vi "Psych Chart Look-up BY HR.vi"(0 "Humidity Ratio [-]":dbl=72.0, 5 "Air Pressure [psia]":dbl=14.7, 7 "1st known value":dbl=55.0, 12 "1st Known Index":u16(ring) items=["DB", "WB", "RH", "HR", "Gr", "Vol", "h", "Dp"]) -> (8 "Output Array":dbl[](array[numeric]))   [LabVIEW 2020]
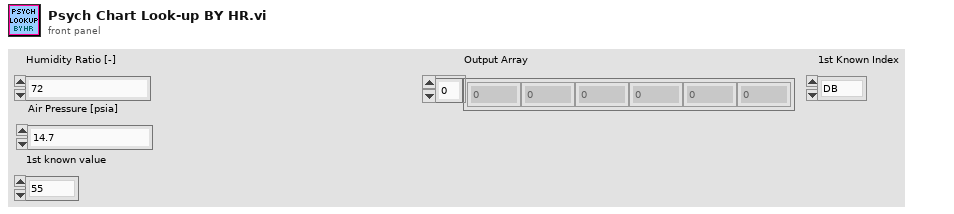
[diagram p1: front panel]
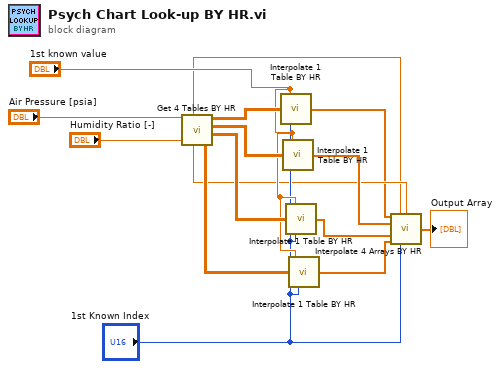
[diagram p0: block diagram]
diagram:
  n1 = call "Get 4 Tables BY HR.vi"("Air Pressure [psia]"="Air Pressure [psia]", "Humidity Ratio [-]"="Humidity Ratio [-]") -> ("Pressure Z"=w5:dbl, "HR Z"=w6:dbl, "HP Higher HR Psych Table"=w13:dbl[][], "HP Lower HR Psych Table"=w12:dbl[][], "LP Higher HR Psych Table"=w11:dbl[][], "LP Lower HR Psych Table"=w10:dbl[][])  [unwired: 1 in]
  n2 = call "Interpolate 1 Table BY HR.vi"("First Known Value"="1st known value", "Psych Table, 1 Press., 1 RH"=w13, "First Known Index"="1st Known Index") -> ("Output Array"=w3:dbl[])  [unwired: 12 in]
  n3 = call "Interpolate 1 Table BY HR.vi"("First Known Value"="1st known value", "Psych Table, 1 Press., 1 RH"=w12, "First Known Index"="1st Known Index") -> ("Output Array"=w9:dbl[])  [unwired: 12 in]
  n4 = call "Interpolate 1 Table BY HR.vi"("First Known Value"="1st known value", "Psych Table, 1 Press., 1 RH"=w11, "First Known Index"="1st Known Index") -> ("Output Array"=w2:dbl[])  [unwired: 12 in]
  n5 = call "Interpolate 1 Table BY HR.vi"("First Known Value"="1st known value", "Psych Table, 1 Press., 1 RH"=w10, "First Known Index"="1st Known Index") -> ("Output Array"=w1:dbl[])  [unwired: 12 in]
  n6 = call "Interpolate 4 Arrays BY HR.vi"("HP Higher HR Array"=w3, "Pressure Z"=w5, "RH Z"=w6, "HP Lower HR Array"=w9, "LP Higher HR Array"=w2, "LP Lower HR Array"=w1, "1st Known Index"="1st Known Index") -> ("Output Array"=→"Output Array":dbl[])  [unwired: 8 in]
